vi "Dynamic Dispatch.Dynamic.vi"() -> ()   [LabVIEW 2016]
uses:
  <vilib>/Platform/TimedLoop/XDataNode/timing_clust.ctl
  <vilib>/Platform/TimedLoop/XDataNode/nitl_modes.ctl
  <vilib>/Platform/TimedLoop/XDataNode/wakeup.ctl
  Classes/Child A/DD Child A.lvclass
  C:/Users/Ryan/Documents/Git/Sourcetree/LabVIEW-Memory-Manager/Source/Tests/Dynamic Dispatch/Classes/Parent/DD Parent.lvclass
  Classes/Child B/DD Child B.lvclass
  <vilib>/platform/TimedLoop/XDataNode/XDataNode.xnode
  Classes/Parent/DD Parent.lvclass
  <vilib>/Platform/TimedLoop/XDataNode/XDNodeRunTimeDep.lvlib
panel:
  out "first iteration":u32
  in  "Iterations":i32=1000
  out "durations":u32[](graph)
  in  "processor":i32=-2
  out "name":string
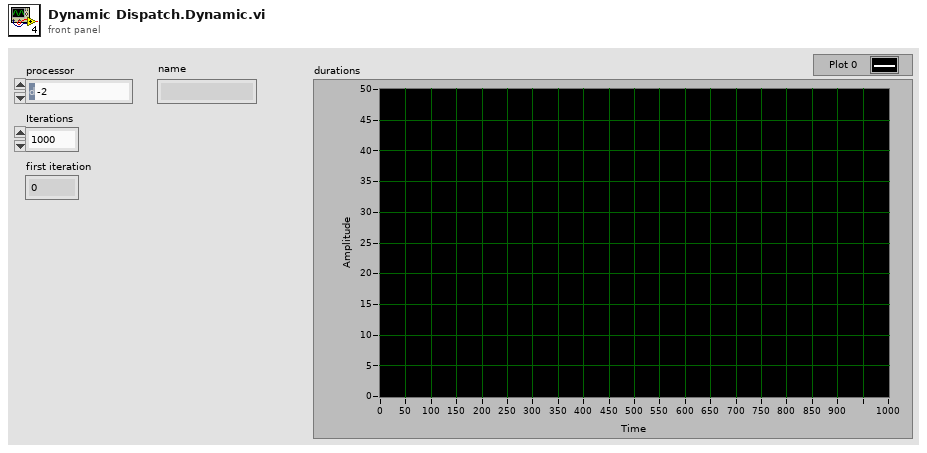
[diagram p1: front panel]
types:
  T1 = typedef "XDNodeRunTimeDep.lvlib/timing_clust.ctl" = cluster{"Expected End [f-1]":u64, "Actual End [f-1]":u64, "Finished Late? [f-1]":bool, "Expected End [i-1]":u64, "Actual End [i-1]":u64, "Finished Late? [i-1]":bool, "Expected Start [i]":u64, "Actual Start [i]":u64, "Expected Start [f]":u64, "Actual Start [f]":u64, "Source Name":string, "Structure Name":string, "Period":i64, "Deadline":i64, "Offset":i64, "Start":i64, "Priority":i32, "Timeout":i32, "Mode":T2, "Wakeup Reason":T3, "Error":errorcluster, "Source Type":string, "Secondary Source Type":string, "Global End Time":u64, "Global Start Time":u64, "Frame Duration":u64, "Iteration Duration":u64, "Assigned CPU":i32, "I/O Scan Engine Mode":u32}
  T2 = typedef "XDNodeRunTimeDep.lvlib/nitl_modes.ctl" = enum32{"No Change", "Process missed periods, maintain original phase", "Discard missed periods, maintain original phase", "Process missed periods, ignore original phase", "Discard missed periods, ignore original phase"}
  T3 = typedef "XDNodeRunTimeDep.lvlib/wakeup.ctl" = enum32{"Normal", "Aborted", "Asynchronous wakeup", "Timing source error", "Timed loop error", "Timeout"}
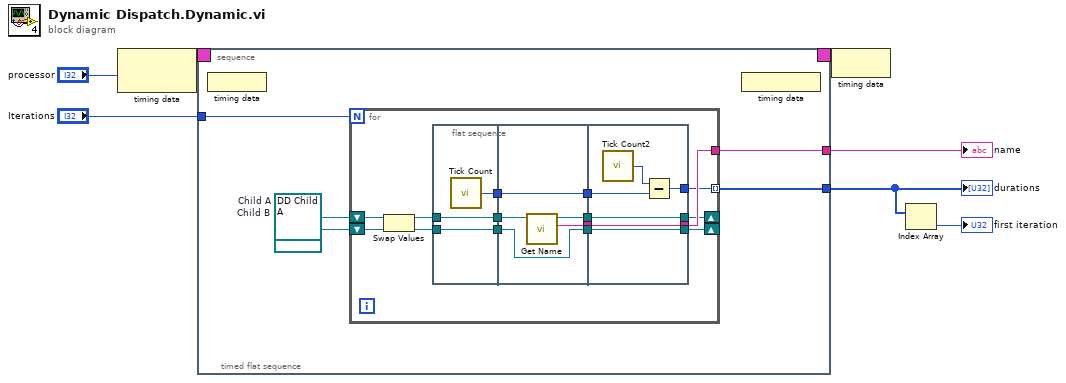
[diagram p0: block diagram]
diagram:
  n1 = node-c288("processor") -> (w7:T1)
  n2 = timed-sequence {
    timing: w7 -> [_]
    timing-out: [_] -> w6
    tunnel: [w10] -> w4
    tunnel: [w9] -> w3
    tunnel: "Iterations" -> [w8]
    n3 = timed-flat-sequence {
      tunnel: [w13] -> w10
      tunnel: [w12] -> w9
      tunnel: w8 -> [w11]
      w15 = refnum<class "DD Child B.lvclass"> refnum  # Child B
      w14 = refnum<class "DD Child A.lvclass"> refnum  # Child A
      n4 = node-c288() -> ()  [unwired: 1 in]
      n5 = for {
        N: w11 -> [_]
        tunnel: [w24] -> w13
        tunnel: [w22] -> w12 mode=indexing
        shift-right: [w23] -> _
        shift-left: w14 -> [w27]
        shift-right: [w19] -> _
        shift-left: w15 -> [w25]
        n6 = Swap Values(12:w27, 14:w25) -> (1:w26:refnum<class "DD Parent.lvclass">, 3:w21:refnum<class "DD Parent.lvclass">)  [unwired: 1 in]
        n7 = flat-sequence {
          tunnel: [w35] -> w32
          tunnel: [w34] -> w29
          tunnel: w26 -> [w34]
          tunnel: w21 -> [w33]
          tunnel: [w33] -> w20
          tunnel: [w40] -> w31
          tunnel: w32 -> [w39]
          tunnel: [w39] -> w30
          tunnel: w29 -> [w38]
          tunnel: [w37] -> w28
          tunnel: w20 -> [w36]
          tunnel: [w36] -> w18
          tunnel: [w46] -> w24
          tunnel: w31 -> [w46]
          tunnel: w30 -> [w45]
          tunnel: [w43] -> w22
          tunnel: w28 -> [w42]
          tunnel: [w42] -> w23
          tunnel: [w41] -> w19
          tunnel: w18 -> [w41]
          frame #0 {
            n8 = call "Tick Count"() -> ("Tick Count(uSec)"=w35:u32)
          }
          frame #1 {
            n9 = call-dynamic "Get Name.vi"("DD Parent in"=w38) -> ("name"=w40:string, "DD Parent out"=w37:refnum<class "DD Parent.lvclass">)  [unwired: 8 in, 1 out]
          }
          frame #2 {
            n10 = call "Tick Count2"() -> ("Tick Count(uSec)"=w44:u32)
            n11 = Subtract(x=w44, y=w45) -> (x-y=w43:u32)
          }
        }
      }
      n12 = node-c288() -> ()  [unwired: 1 out]
    }
  }
  "name" <- w4
  "durations" <- w3
  n13 = node-c288(w6) -> ()
  n14 = Index Array(array=w3) -> (element=→"first iteration":u32)  [unwired: 1 in]
